vi "MRC Allocate String Array.vi"(8 "error in (no error)":errorcluster, 10 "length":i64, 11 "mrcStringArray":cluster{"str":u64, "len":i64}) -> (0 "error out":errorcluster)   [LabVIEW 2026, in "MrcLib.lvlib"]
doc: "void MRC_CALLCONV MRC_FreeStringArray(const struct MRC_String* mrcStringArray,\n size_t length);"
uses:
  MrcLib.lvlib
  MrcLib.dll
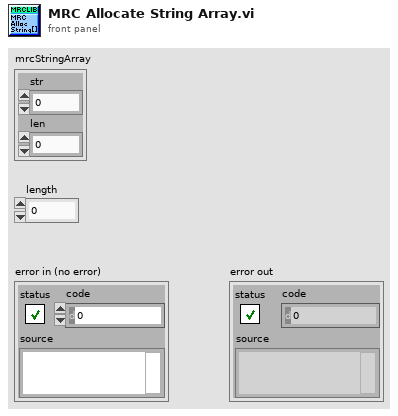
[diagram p1: front panel]
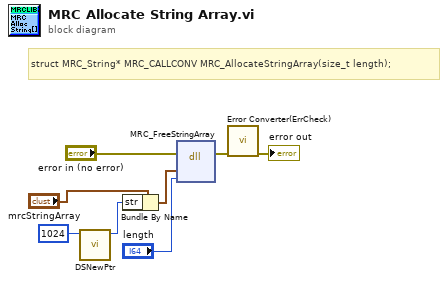
[diagram p0: block diagram]
diagram:
  # "struct MRC_String* MRC_CALLCONV MRC_AllocateStringArray(size_t length);"
  n1 = call <vilib>:"DSNewPtr.vi"("Size"=u64 1024) -> ("Pointer"=w6:u64)  [unwired: 9 in, 1 out]
  n2 = Bundle By Name(cluster="mrcStringArray", "str"=w6) -> (w5:cluster{"str":u64, "len":i64})
  n3 = dll-call lib="MrcLib.*" fn="MRC_FreeStringArray"(error in="error in (no error)", "mrcStringArray"=w5, "length"="length") -> (error out=w2:errorcluster)  [unwired: 5 in, 1 out]
  n4 = call <vilib>:"Error Converter(ErrCheck).vi"("error in (no error)"=w2) -> ("error out"=→"error out":errorcluster)  [unwired: 10 in]
